vi "PXI Nest Control.vi"(3 "error in (no error)":errorcluster {"code" format="%.0x"}, 4 "Enum":T1(ring), 5 "SetValue":dbl format="%0.2f") -> (0 "error out":errorcluster, 1 "Measure":dbl format="%0.2f", 2 "Bool":bool)   [LabVIEW 2014]
uses:
  <vilib>/DAQmx/read.llb/DAQmx Read (Analog DBL 1Chan 1Samp).vi
  <vilib>/DAQmx/write.llb/DAQmx Write (Analog DBL 1Chan 1Samp).vi
  <vilib>/DAQmx/read.llb/DAQmx Read (Digital Bool 1Line 1Point).vi
  <vilib>/DAQmx/miscellaneous.llb/DAQmx Fill In Error Info.vi
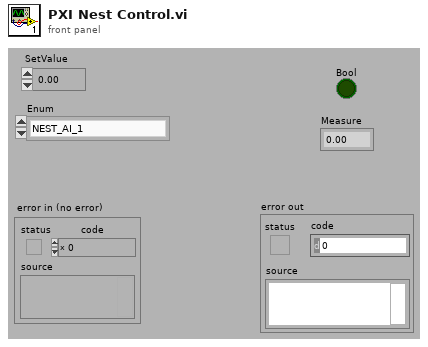
[diagram p1: front panel]
types:
  T1 = enum16{"NEST_AI_1", "NEST_A1_2", "NEST_AI_3", "NEST_AI_4", "NEST_AI_5", "NEST_AI_6", "NEST_A0_1", "NEST_A0_2", "NEST_DI_1", "NEST_DI_2", "NEST_DI_3"}
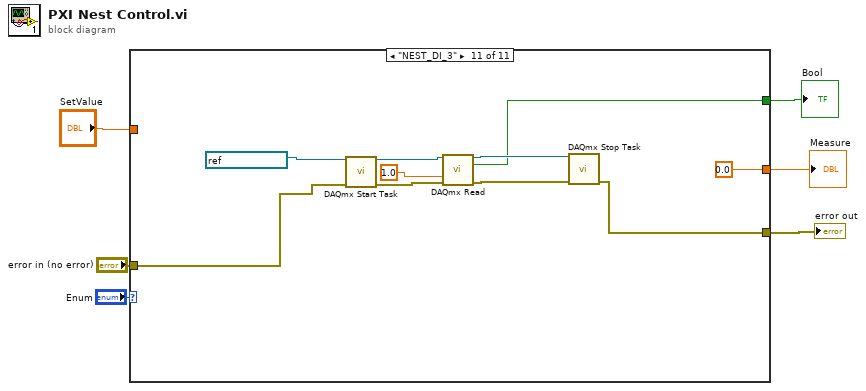
[diagram p0: block diagram]
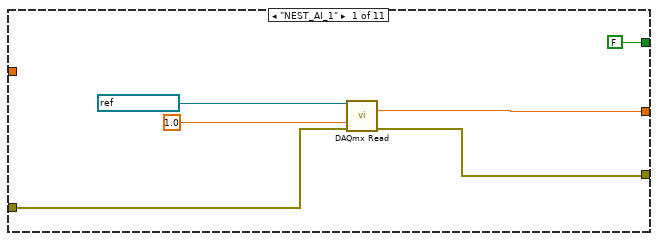
[diagram p2: hidden frame]
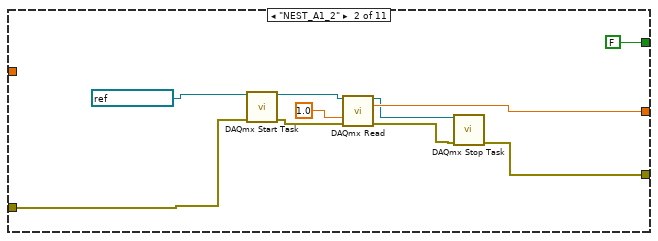
[diagram p3: hidden frame]
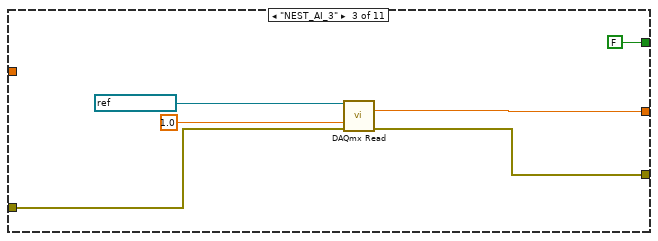
[diagram p4: hidden frame]
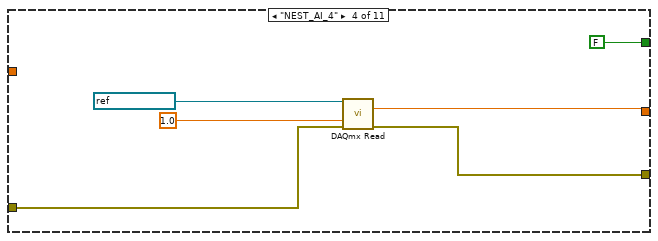
[diagram p5: hidden frame]
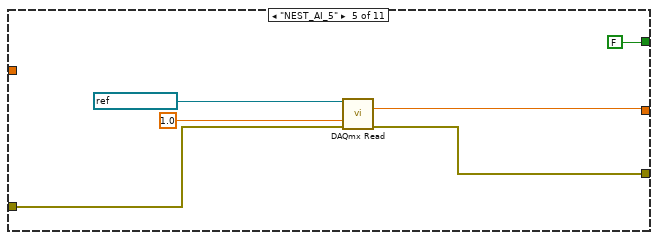
[diagram p6: hidden frame]
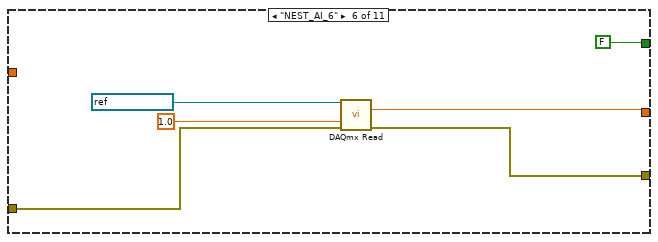
[diagram p7: hidden frame]
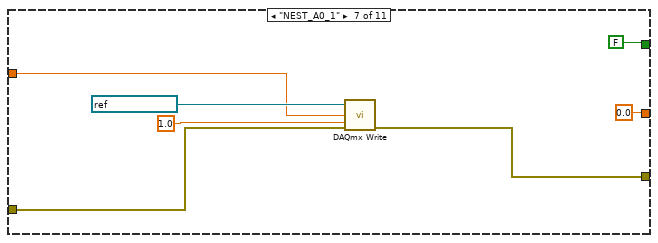
[diagram p8: hidden frame]
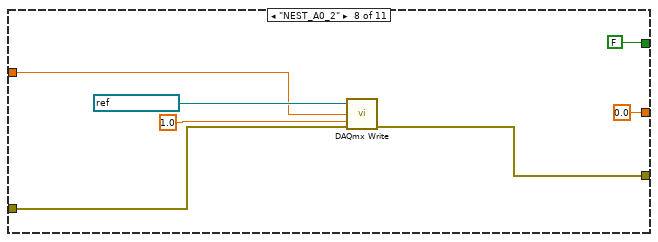
[diagram p9: hidden frame]
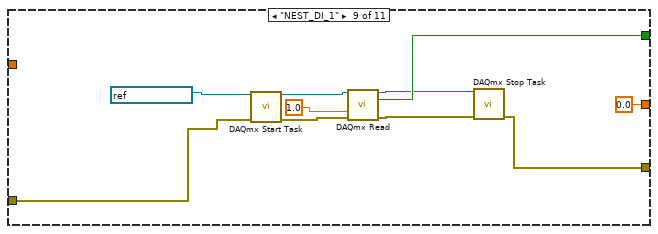
[diagram p10: hidden frame]
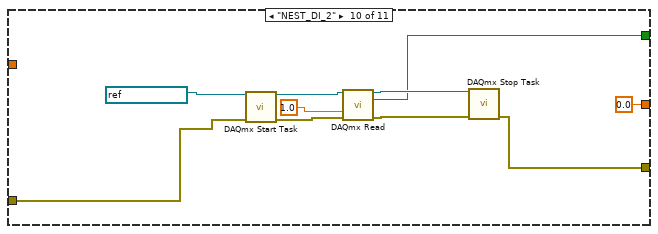
[diagram p11: hidden frame]
diagram:
  n1 = case shown="\"NEST_DI_3\"" "Enum" {
    tunnel: [w8 w14 w25 w31 w37 w43 w49 w56 w61 w72 w83] -> w5
    tunnel: "error in (no error)" -> [w11 w18 w24 w30 w36 w44 w51 w58 w65 w73 w84]
    tunnel: [w9 w22 w26 w32 w38 w42 0.0 ("data") 0.0 ("data") 0.0 ("data") 0.0 ("data") 0.0 ("data")] -> w3
    tunnel: "SetValue" -> [_ _ _ _ _ _ w50 w57 _ _ _]
    tunnel: [FALSE ("data") FALSE ("data") FALSE ("data") FALSE ("data") FALSE ("data") FALSE ("data") FALSE ("data") FALSE ("data") w69 w71 w82] -> w1
    frame "NEST_AI_1" {
      n2 = call-poly <vilib>:"DAQmx Read.vi"("task/channels in"=refnum<k21> "NEST_AI_1", "timeout"=1.0, "error in"=w11) -> ("data"=w9:dbl, "error out"=w8:errorcluster)  [unwired: 10 in, 1 out]
    }
    frame "NEST_A1_2" {
      n3 = call <vilib>:"DAQmx Start Task.vi"("task/channels in"=refnum<k21> "NEST_AI_2", "error in"=w18) -> ("task out"=w16:refnum<k21>, "error out"=w19:errorcluster)  [unwired: 12 in]
      n4 = call-poly <vilib>:"DAQmx Read.vi"("task/channels in"=w16, "timeout"=1.0, "error in"=w19) -> ("task out"=w13:refnum<k21>, "data"=w22:dbl, "error out"=w15:errorcluster)  [unwired: 10 in]
      n5 = call <vilib>:"DAQmx Stop Task.vi"("task/channels in"=w13, "error in"=w15) -> ("error out"=w14:errorcluster)  [unwired: 12 in, 1 out]
    }
    frame "NEST_AI_3" {
      n6 = call-poly <vilib>:"DAQmx Read.vi"("task/channels in"=refnum<k21> "NEST_AI_3", "timeout"=1.0, "error in"=w24) -> ("data"=w26:dbl, "error out"=w25:errorcluster)  [unwired: 10 in, 1 out]
    }
    frame "NEST_AI_4" {
      n7 = call-poly <vilib>:"DAQmx Read.vi"("task/channels in"=refnum<k21> "NEST_AI_4", "timeout"=1.0, "error in"=w30) -> ("data"=w32:dbl, "error out"=w31:errorcluster)  [unwired: 10 in, 1 out]
    }
    frame "NEST_AI_5" {
      n8 = call-poly <vilib>:"DAQmx Read.vi"("task/channels in"=refnum<k21> "NEST_A1_5", "timeout"=1.0, "error in"=w36) -> ("data"=w38:dbl, "error out"=w37:errorcluster)  [unwired: 10 in, 1 out]
    }
    frame "NEST_AI_6" {
      n9 = call-poly <vilib>:"DAQmx Read.vi"("task/channels in"=refnum<k21> "NEST_AI_6", "timeout"=1.0, "error in"=w44) -> ("data"=w42:dbl, "error out"=w43:errorcluster)  [unwired: 10 in, 1 out]
    }
    frame "NEST_A0_1" {
      n10 = call-poly <vilib>:"DAQmx Write.vi"("task/channels in"=refnum<k21> "NEST_AO_1", "data"=w50, "timeout"=1.0, "error in"=w51) -> ("error out"=w49:errorcluster)  [unwired: 9 in, 2 out]
    }
    frame "NEST_A0_2" {
      n11 = call-poly <vilib>:"DAQmx Write.vi"("task/channels in"=refnum<k21> "NEST_AO_2", "data"=w57, "timeout"=1.0, "error in"=w58) -> ("error out"=w56:errorcluster)  [unwired: 9 in, 2 out]
    }
    frame "NEST_DI_1" {
      n12 = call <vilib>:"DAQmx Start Task.vi"("task/channels in"=refnum<k21> "NEST_DI_1", "error in"=w65) -> ("task out"=w66:refnum<k21>, "error out"=w64:errorcluster)  [unwired: 12 in]
      n13 = call-poly <vilib>:"DAQmx Read.vi"("task/channels in"=w66, "timeout"=1.0, "error in"=w64) -> ("task out"=w63:refnum<k21>, "data"=w69:bool, "error out"=w62:errorcluster)  [unwired: 10 in]
      n14 = call <vilib>:"DAQmx Stop Task.vi"("task/channels in"=w63, "error in"=w62) -> ("error out"=w61:errorcluster)  [unwired: 12 in, 1 out]
    }
    frame "NEST_DI_2" {
      n15 = call <vilib>:"DAQmx Start Task.vi"("task/channels in"=refnum<k21> "NEST_DI_2", "error in"=w73) -> ("task out"=w76:refnum<k21>, "error out"=w77:errorcluster)  [unwired: 12 in]
      n16 = call-poly <vilib>:"DAQmx Read.vi"("task/channels in"=w76, "timeout"=1.0, "error in"=w77) -> ("task out"=w78:refnum<k21>, "data"=w71:bool, "error out"=w79:errorcluster)  [unwired: 10 in]
      n17 = call <vilib>:"DAQmx Stop Task.vi"("task/channels in"=w78, "error in"=w79) -> ("error out"=w72:errorcluster)  [unwired: 12 in, 1 out]
    }
    frame "NEST_DI_3" {
      n18 = call <vilib>:"DAQmx Start Task.vi"("task/channels in"=refnum<k21> "NEST_DI_3", "error in"=w84) -> ("task out"=w87:refnum<k21>, "error out"=w88:errorcluster)  [unwired: 12 in]
      n19 = call-poly <vilib>:"DAQmx Read.vi"("task/channels in"=w87, "timeout"=1.0, "error in"=w88) -> ("task out"=w89:refnum<k21>, "data"=w82:bool, "error out"=w90:errorcluster)  [unwired: 10 in]
      n20 = call <vilib>:"DAQmx Stop Task.vi"("task/channels in"=w89, "error in"=w90) -> ("error out"=w83:errorcluster)  [unwired: 12 in, 1 out]
    }
  }
  "error out" <- w5
  "Measure" <- w3
  "Bool" <- w1
